vi "Agilent ESG_Open.vi"(8 "error in":errorcluster, 10 "Reset?":bool=TRUE, 11 "Alias":string) -> (0 "error out":errorcluster {"code" format="%.0x"}, 3 "Handle":variant)   [LabVIEW 2015]
uses:
  <instrlib>/Agilent ESG Series/Agilent ESG Series.lvlib
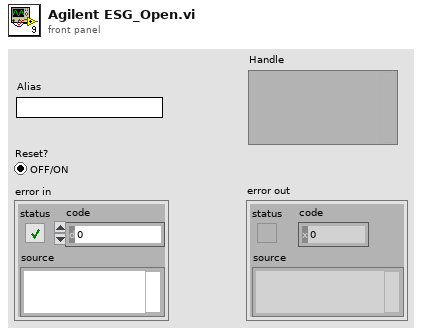
[diagram p1: front panel]
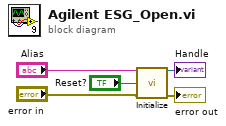
[diagram p0: block diagram]
diagram:
  n1 = call <instrlib>:"Initialize.vi"("VISA Resource Name"="Alias", "Reset? (T: Yes)"="Reset?", "error in (no error)"="error in") -> ("VISA Resource Name Out"=→"Handle":refnum<visa-resource-name>, "error out"=→"error out":errorcluster)  [unwired: 11 in]
